vi "Joystick and Camera.vi"() -> ()   [LabVIEW 2020]
uses:
  Classes/Controller/Camera/Camera.lvclass
  Classes/Controller/Controller.lvclass
  Classes/Controller/I-O/I-O.lvclass
  Classes/Controller/Motion/A3200/A3200.lvclass
  Classes/Controller/Motion/Motion.lvclass
  Classes/Controller/Camera/Machine Vision.ctl
  Classes/Controller/Camera/Camera settings.ctl
  Classes/Controller/Camera/Image processing.ctl
  Classes/Controller/Camera/Material.ctl
panel:
  in  "Find fiducial":bool
  in  "Loop count":dbl=1.0
  in  "X, Y pixel stride":dbl[](array[numeric])=[1520.0, 2160.0]
  in  "Draw spiral":bool
  out "Move by":dbl[](array[numeric])
  in  "Find in Image":bool
  in  "Screen Grab":bool
  in  "Focus step size":dbl format="%#_13g"
  in  "number of focus steps":i32
  out "Radius (Real-World)":dbl
  out "error out":errorcluster
  in  "Find fiducial center":bool
  out "Average Strength":dbl
  in  "Focus":bool
  in  "Material":T1
  in  "Override presets":bool
  in  "Camera settings":T2={"Gamma"=1.6, "Gain"=0, "Sharpness"=0, "Contrast"=0.0, "Exposure"=0.0078125} {"Exposure" min=0.000244140625 max=0.5 scale=0.0002..0.5; "Contrast" min=0.0 max=1.0 scale=0.0..1.0; "Sharpness" min=0 max=2 step=1 scale=0.0..2.0; "Gain" min=0 max=100 step=1 scale=0.0..100.0; "Gamma" min=0.01 max=10.0 scale=0.01..10.0}
  in  "Image processing":T3={"Brightness"=128.0, "Contrast"=45.0, "Gamma"=1.0471123} {"Brightness" scale=0.0..400.0; "Contrast" scale=0.0..90.0; "Gamma" scale=0.005..5.0}
  out "XYZTheta Out":dbl[](array[numeric])
  in  "Machine Vision":T4
  in  "Move 10cm Right":bool
  in  "Move 10cm Backward":bool
  in  "Move 10cm Forward":bool
  in  "Move 10cm Left":bool
  in  "Record Measurement":bool=TRUE
  in  "Dismount Silicon Tray":bool
  in  "Secure Silicon Tray":bool
  in  "Z Go":bool
  in  "Position":dbl
  in  "XYZTheta":dbl[](array[numeric])
  in  "Go":bool
  in  "Joystick":bool
  out "Sum":dbl[](array[numeric]) format="%#.6g"
  out "Gantry":dbl[](array[numeric]) format="%#.6g"
  in  "Stop":bool
  out "Image":T5(plugin-control)
  out "Camera":dbl[](array[numeric])
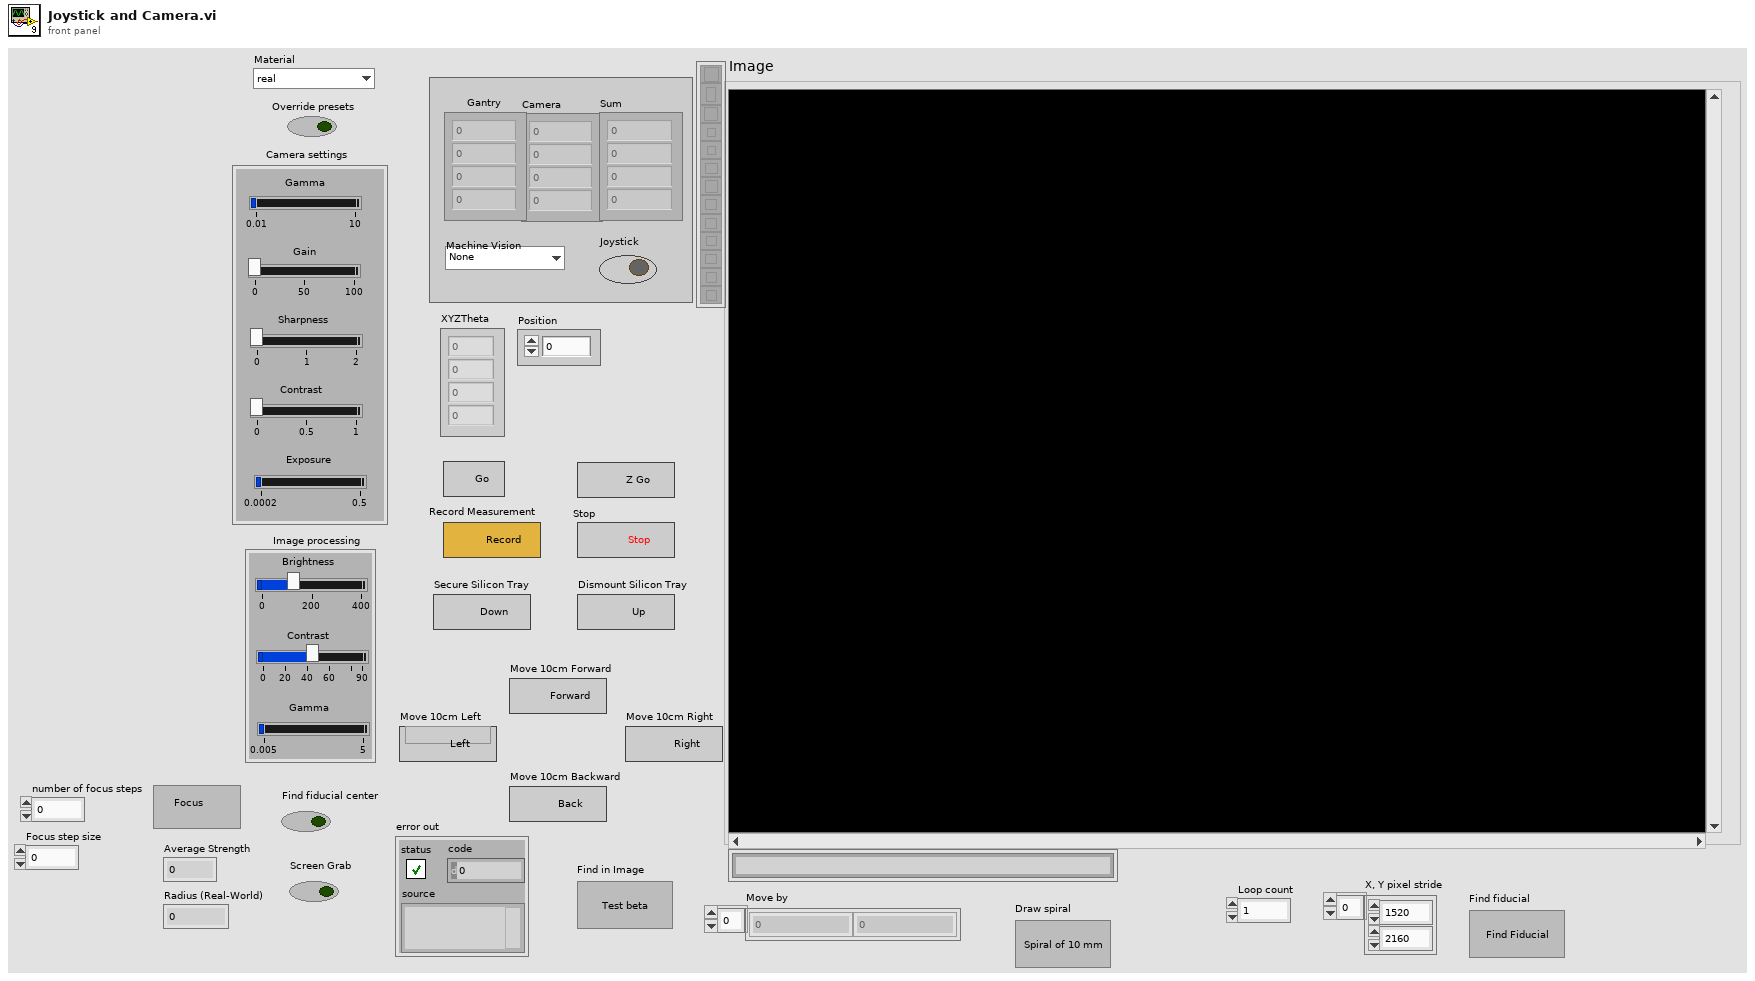
[diagram p1: front panel]
types:
  T1 = typedef "Camera.lvclass/Material.ctl" = enum16{"real", "dummy", "PETG"}
  T2 = typedef "Camera.lvclass/Camera settings.ctl" = cluster{"Gamma":dbl, "Gain":i64, "Sharpness":i64, "Contrast":dbl, "Exposure":dbl}
  T3 = typedef "Camera.lvclass/Image processing.ctl" = cluster{"Brightness":sgl, "Contrast":sgl, "Gamma":sgl}
  T4 = typedef "Camera.lvclass/Machine Vision.ctl" = enum16{"None", "Tray Fiducials", "HPK Silicon", "100um dot", "Hexaboard", "Corner (TL, BR)", "Corner (BL, TR)", "BP gold pad 1", "BP gold pad 2", "BP gold pad 3", "dummy sensor CH2", "dummy sensor CH7", "dummy sensor CH191", "dummy sensor CH197", "sensor box", "sensor circle", "PCB PETG CH2", "PCB PETG CH7", "PCB PETG CH191", "PCB PETG CH197"}
  T5 = typedef "IMAQ Image.ctl" = refnum<image>
  T6 = enum16{"open", "replace", "create", "open or create", "replace or create", "replace or create with confirmation"}
  T7 = typedef "Controller.lvclass/Controllers.ctl" = cluster{"I-O.lvclass":refnum<class "I-O.lvclass">, "Gantry":refnum<k24>, "Dispenser":refnum<visa-resource-name>}
  T8 = typedef "I-O.lvclass/Pin Map.ctl" = cluster{"Region Valves":i32[], "Extra Valves":dbl[][][], "Tool Primary Valve":i32, "Tool Secondary Valve":i32, "Region Sensors":i32[], "Extra Sensors":dbl[][][], "Tool Primary Sensor":dbl, "Tool Secondary Sensor":dbl, "Compression Sensor":dbl, "5V":i32, "Dispenser Sensor":dbl}
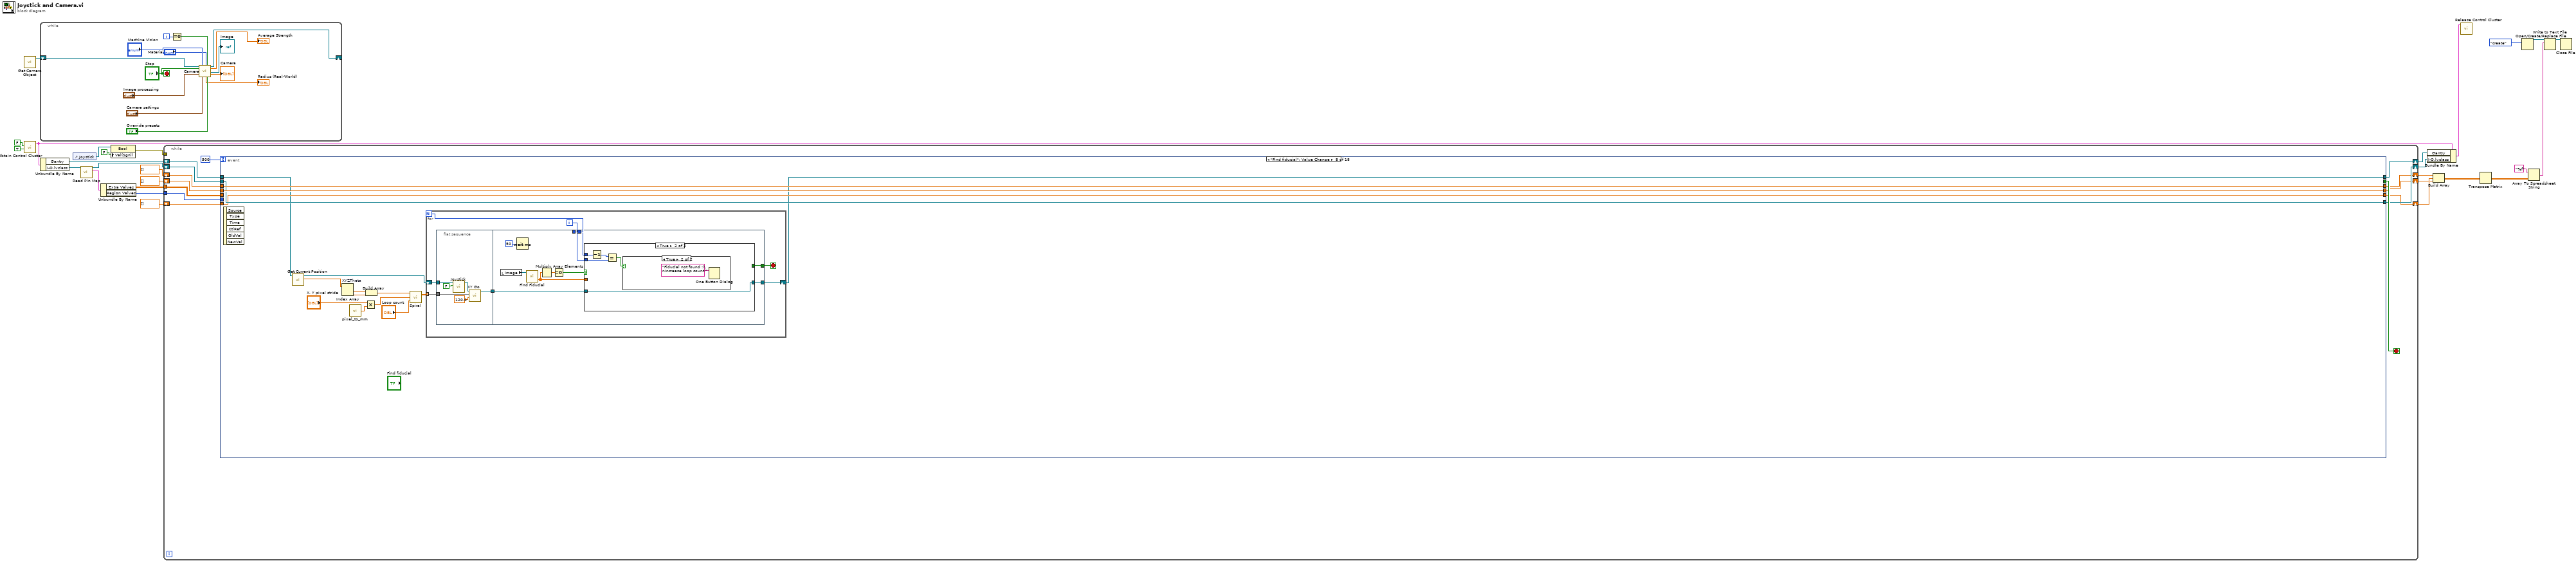
[diagram p0: block diagram]
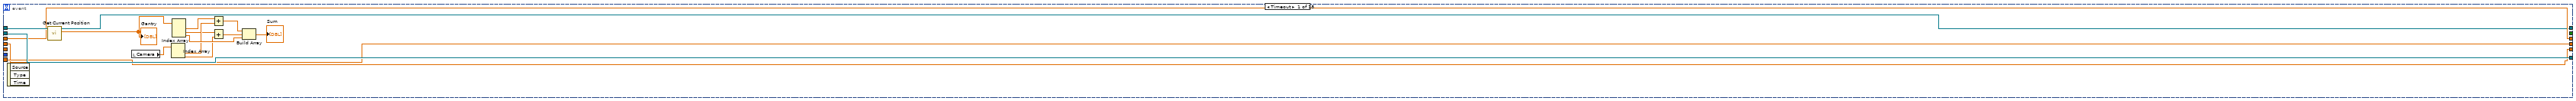
[diagram p2: hidden frame]
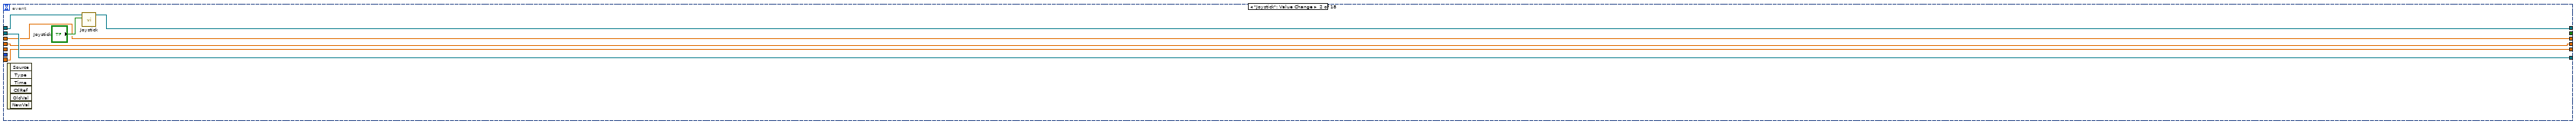
[diagram p3: hidden frame]
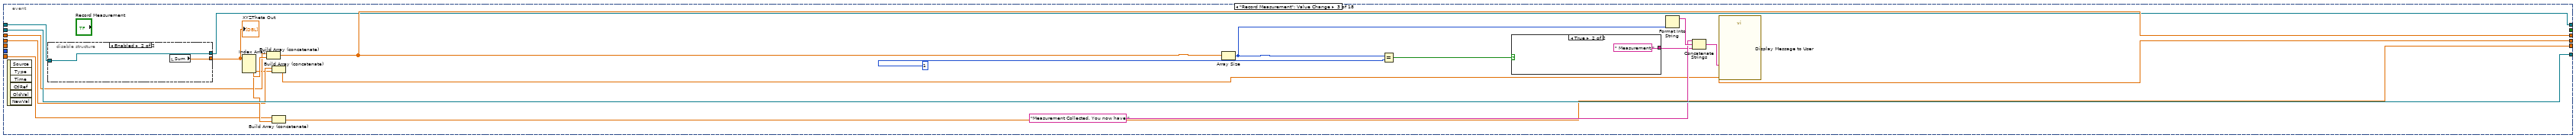
[diagram p4: hidden frame]
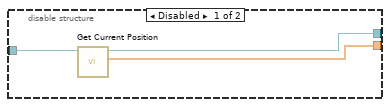
[diagram p5: hidden frame]
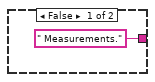
[diagram p6: hidden frame]
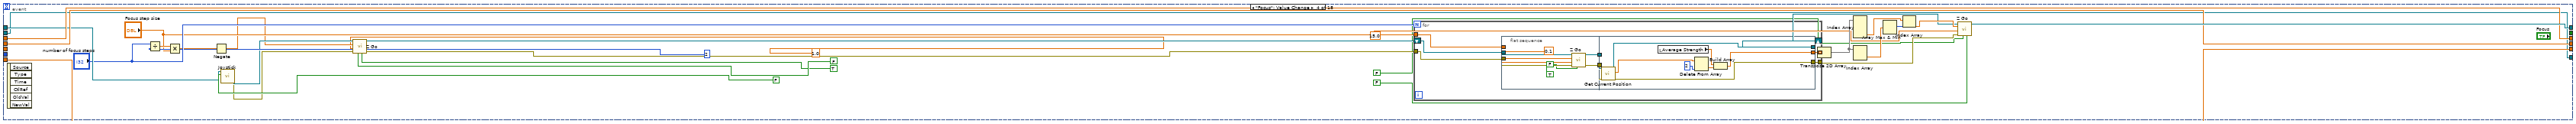
[diagram p7: hidden frame]
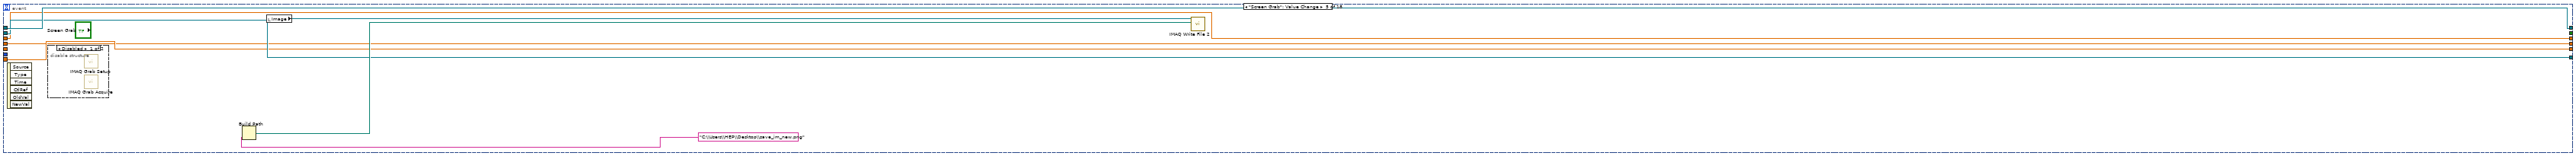
[diagram p8: hidden frame]
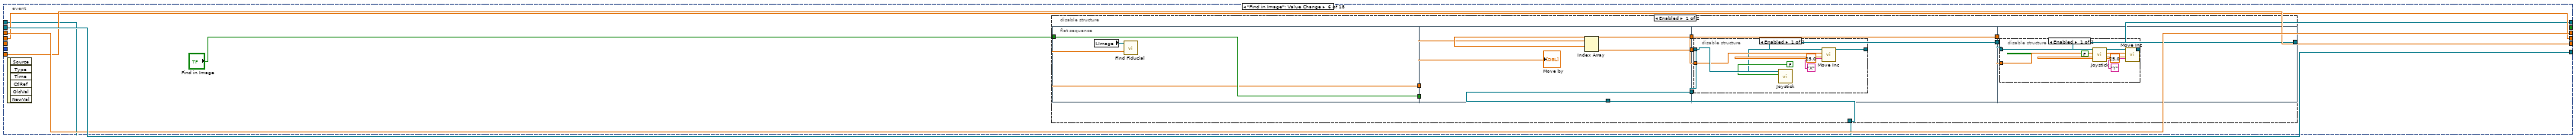
[diagram p10: hidden frame]
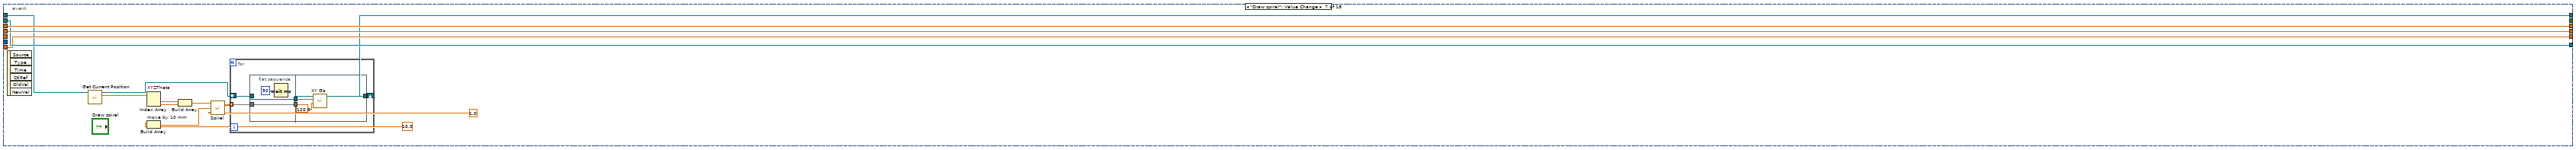
[diagram p14: hidden frame]
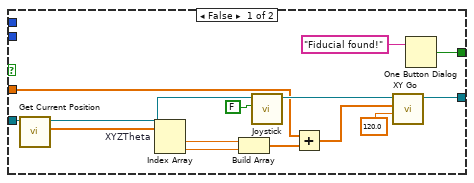
[diagram p15: hidden frame]
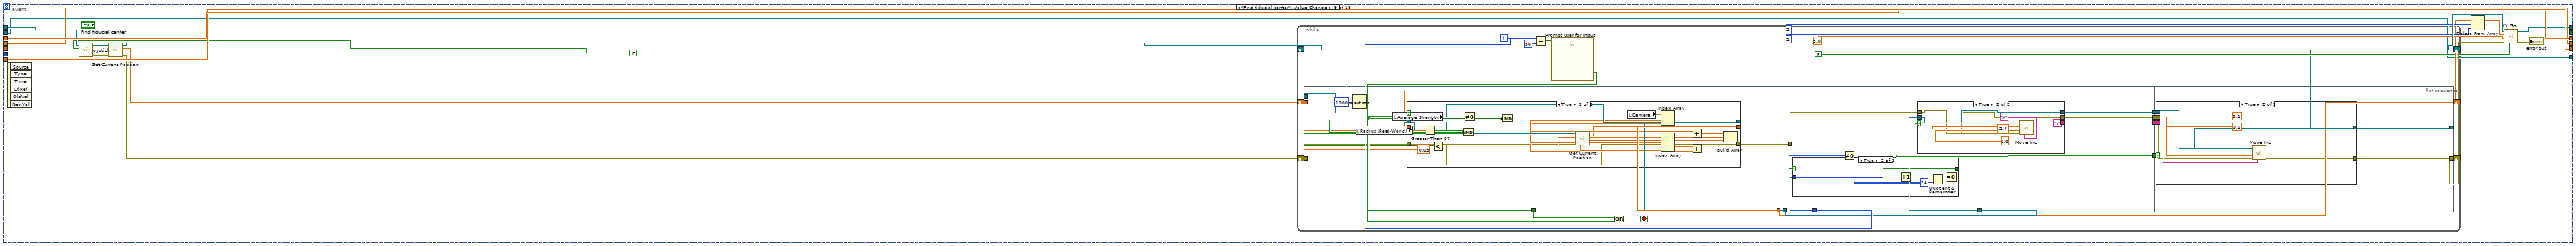
[diagram p17: hidden frame]
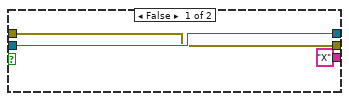
[diagram p20: hidden frame]
diagram:
  n1 = call "Get Camera Object.vi"() -> ("Camera out"=w23:refnum<class "Camera.lvclass">)  [unwired: 10 in, 1 out]
  n2 = call "Obtain Control Cluster.vi"("I/O"=TRUE, "Dispense"=FALSE) -> ("Control Out"=w1:T7)  [unwired: 9 in]
  n3 = while {
    shift-right: [w42] -> _
    shift-left: w23 -> [w43]
    i -> [w34]
    stop <- "Stop" stop-if-true
    n4 = Equal To 0?(x=w34) -> (x = 0?=w33:bool)
    n5 = call "Camera.vi"("Camera in"=w43, "Stop"="Stop", "BCG Image Processing"="Image processing", "Machine Vision"="Machine Vision", "Camera settings"="Camera settings", "Material"="Material", "Loop 0"=w33, "Override presets"="Override presets") -> ("Radius (Real-World)"=→"Radius (Real-World)":dbl, "Camera out"=w42:refnum<class "Camera.lvclass">, "Average Strength"=→"Average Strength":dbl, "Image"=→"Image":T5, "Camera"=→"Camera":dbl[])  [unwired: 6 in, 1 out]
  }
  n6 = Unbundle By Name(w1) -> ("Gantry"=w24:refnum<k24>, "I-O.lvclass"=w22:refnum<class "I-O.lvclass">)
  n7 = control-ref of="Joystick"() -> (w28:refnum<vi>)
  n8 = call-dynamic "Read Pin Map.vi"("I-O in"=w22) -> ("Pin Map 2"=w20:T8, "I-O out"=w21:refnum<class "I-O.lvclass">)  [unwired: 8 in, 1 out]
  n9 = Unbundle By Name(w20) -> ("Extra Valves"=w18:dbl[][][], "Region Valves"=w19:i32[])
  n10 = property class="Bool"(reference=w28, "Val(Sgnl)"=FALSE ("Value (Signaling)")) -> (error out=w27:errorcluster)  [unwired: 1 in, 1 out]
  n11 = while {
    shift-right: [w44] -> w4
    shift-left: w24 -> [w55]
    tunnel: w27 -> [_]
    shift-right: [w53] -> w3
    shift-left: w21 -> [w54]
    tunnel: w19 -> [w52]
    tunnel: w18 -> [w51]
    shift-right: [w46] -> w6
    shift-left: dbl[] [] -> [w50]
    shift-right: [w48] -> w7
    shift-left: dbl[] [] -> [w49]
    shift-right: [w45] -> w8
    shift-left: dbl[] [] -> [w47]
    stop <- w56 stop-if-true
    n12 = event shown="[7] \"Find fiducial\": Value Change" {
      selector: _ -> [_ _ _ _ _ _ _ _ _ _ _ _ _ _ _ _ _ _]
      dyn-events: _ -> [_ _ _ _ _ _ _ _ _ _ _ _ _ _ _ _ _ _]
      timeout: 500 -> [_ _ _ _ _ _ _ _ _ _ _ _ _ _ _ _ _ _]
      tunnel: [_ _ _ _ _ _ _ _ _ _ _ _ _ _ _ _ _ TRUE] -> w56
      tunnel: w55 -> [w73 w80 w83 w124 w169 w174 w228 w257 w323 w442 w453 w464 w475 w477 w487 w504 w523 w531]
      tunnel: w54 -> [w72 w78 w100 w108 w168 w178 w231 w260 w306 w437 w449 w461 w472 w484 w496 w501 w520 w529]
      tunnel: [w72 w78 w100 w108 w168 w178 w231 w260 w306 w437 w449 w461 w472 w481 w491 w501 w520 w529] -> w53
      tunnel: w52 -> [_ _ _ _ _ _ _ _ _ _ _ _ _ w486 w495 _ _ _]
      tunnel: w51 -> [_ _ _ _ _ _ _ _ _ _ _ _ _ _ _ _ _ _]
      tunnel: w50 -> [w71 w77 w87 w127 w166 w176 w230 w259 w325 w440 w452 w463 w474 w480 w490 w500 w519 w528]
      tunnel: [w71 w77 w91 w127 w166 w176 w230 w259 w325 w440 w452 w463 w474 w480 w490 w500 w519 w528] -> w46
      tunnel: w49 -> [w70 w76 w88 w128 w167 w177 w233 w262 w326 w439 w451 w462 w473 w479 w489 w499 w518 w527]
      tunnel: [w70 w76 w90 w128 w167 w177 w233 w262 w326 w439 w451 w462 w473 w479 w489 w499 w518 w527] -> w48
      tunnel: w47 -> [w69 w75 w86 w126 w165 w175 w232 w261 w324 w438 w450 w460 w471 w478 w488 w498 w517 w526]
      tunnel: [w69 w75 w84 w126 w165 w175 w232 w261 w324 w438 w450 w460 w471 w478 w488 w498 w517 w526] -> w45
      tunnel: [w68 w74 w81 w129 w169 w173 w229 w258 w320 w436 w445 w455 w467 w477 w487 w497 w516 w524] -> w44
      event Timeout {
        n13 = event-data() -> ()  [unwired: 1 in, 3 out]
        n14 = call "Get Current Position.vi"("Gantry In"=w73) -> ("XYZTheta Out"=w65:dbl[], "Gantry Out"=w68:refnum<k24>)  [unwired: 8 in, 1 out]
        "Gantry" <- w65
        n15 = local read "Camera"() -> (w62:dbl[])
        n16 = Index Array(array=w62) -> (element #1=w61:dbl, element #2=w58:dbl)  [unwired: 2 in]
        n17 = Index Array(array=w65) -> (element #1=w63:dbl, element #2=w59:dbl, element #3=w66:dbl)  [unwired: 3 in]
        n18 = Add(x=w63, y=w61) -> (x+y=w64:dbl)
        n19 = Add(x=w59, y=w58) -> (x+y=w60:dbl)
        n20 = Build Array(w64, w60, w66) -> (→"Sum":dbl[])
      }
      event "Joystick": Value Change {
        n21 = event-data() -> ()  [unwired: 1 in, 6 out]
        n22 = call "Joystick.vi"("Joystick"="Joystick", "Gantry In"=w80) -> ("Gantry Out"=w74:refnum<k24>)  [unwired: 8 in, 1 out]
      }
      event "Record Measurement": Value Change {
        n23 = event-data() -> ()  [unwired: 1 in, 6 out]
        n24 = disable-structure shown="Enabled" {
          disable-tunnel: [w102 w104] -> w82
          disable-tunnel: w83 -> [w103 w105]
          disable-tunnel: [w101 w105] -> w81
          frame Disabled {
            n25 = call "Get Current Position.vi"("Gantry In"=w103) -> ("XYZTheta Out"=w102:dbl[], "Gantry Out"=w101:refnum<k24>)  [unwired: 8 in, 1 out]
          }
          frame Enabled {
            n26 = local read "Sum"() -> (w104:dbl[])
          }
        }
        "XYZTheta Out" <- w82
        n27 = Index Array(array=w82) -> (element #1=w99:dbl, element #2=w89:dbl, element #3=w85:dbl)  [unwired: 3 in]
        n28 = Build Array (concatenate) "Build Array"(w88, w99) -> (w90:dbl[])
        n29 = Build Array (concatenate)(w86, w85) -> (w84:dbl[])
        n30 = Build Array (concatenate)(w87, w89) -> (w91:dbl[])
        n31 = Array Size(array=w90) -> (size(s)=w94:i32)
        n32 = Equal?(x=w94, y=1) -> (x = y?=w93:bool)
        n33 = case shown="True" w93 {
          tunnel: [" Measurements." " Measurement."] -> w92
          frame False {
          }
          frame True {
          }
        }
        n34 = Format Into String(w94) -> (resulting string=w98:string)  [unwired: 3 in, 1 out]
        n35 = Concatenate Strings("Measurement Collected. You now have ", w98, w92) -> (w96:string)
        n36 = call "Display Message to User"("Message"=w96) -> ()  [unwired: 9 in, 2 out]
      }
      event "Focus": Value Change {
        n37 = event-data() -> ()  [unwired: 1 in, 6 out]
        n38 = Divide(x="number of focus steps", y=2) -> (x/y=w121:dbl)
        n39 = Multiply(x=w121, y="Focus step size") -> (x*y=w119:dbl)
        n40 = Negate(x=w119) -> (-x=w114:dbl)
        n41 = call "Joystick.vi"("Joystick"=FALSE, "Gantry In"=w124) -> ("error out"=w115:errorcluster, "Gantry Out"=w118:refnum<k24>)  [unwired: 8 in]
        n42 = call "Z Go.vi"("Increment"=TRUE, "Return Immediately"=FALSE ("Increment"), "error in (no error)"=w115, "Speed In"=1.0 ("Speed"), "Position In"=w114, "Gantry In"=w118) -> ("error out"=w116:errorcluster, "Gantry Out"=w117:refnum<k24>)  [unwired: 2 in, 2 out]
        n43 = for {
          N: "number of focus steps" -> [_]
          tunnel: [w143] -> w137 mode=indexing
          tunnel: w116 -> [w142]
          tunnel: [w140] -> w130
          shift-right: [w144] -> w131
          shift-left: w117 -> [w146]
          tunnel: "Focus step size" -> [w139]
          n44 = flat-sequence {
            tunnel: w146 -> [w153]
            tunnel: [w152] -> w145
            tunnel: w142 -> [w151]
            tunnel: [w150] -> w141
            tunnel: w139 -> [w149]
            tunnel: w145 -> [w163]
            tunnel: [w162] -> w144
            tunnel: [w161] -> w143
            tunnel: w141 -> [w157]
            tunnel: [w156] -> w140
            frame #0 {
              n45 = call "Z Go.vi"("Increment"=TRUE, "Return Immediately"=FALSE ("Increment"), "error in (no error)"=w151, "Speed In"=0.1 ("Speed"), "Position In"=w149, "Gantry In"=w153) -> ("error out"=w150:errorcluster, "Gantry Out"=w152:refnum<k24>)  [unwired: 2 in, 2 out]
            }
            frame #1 {
              n46 = call "Get Current Position.vi"("error in (no error)"=w157, "Gantry In"=w163) -> ("error out"=w156:errorcluster, "XYZTheta Out"=w160:dbl[], "Gantry Out"=w162:refnum<k24>)  [unwired: 7 in]
              n47 = local read "Average Strength"() -> (w155:dbl)
              n48 = Delete From Array(array=w160, index=2) -> (deleted portion=w158:dbl)  [unwired: 1 in, 1 out]
              n49 = Build Array(w155, w158) -> (w161:dbl[])
            }
          }
        }
        n50 = Transpose 2D Array(2D array=w137) -> (transposed array=w136:dbl[][])
        n51 = Index Array(array=w136) -> (element #2=w135:dbl[])  [unwired: 4 in, 1 out]
        n52 = Index Array(array=w136) -> (element=w138:dbl[])  [unwired: 2 in]
        n53 = Array Max & Min(array=w138) -> (max index (indices)=w134:i32)  [unwired: 3 out]
        n54 = Index Array(array=w135, index=w134) -> (element=w133:dbl)
        n55 = call "Z Go.vi"("Increment"=FALSE, "Return Immediately"=FALSE ("Increment"), "error in (no error)"=w130, "Speed In"=15.0 ("Speed"), "Position In"=w133, "Gantry In"=w131) -> ("Gantry Out"=w129:refnum<k24>)  [unwired: 2 in, 3 out]
      }
      event "Screen Grab": Value Change {
        n56 = event-data() -> ()  [unwired: 1 in, 6 out]
        n57 = disable-structure shown="Disabled" {
          frame Disabled {
            n58 = call <vilib>:"IMAQ Grab Setup.vi"() -> ()  [unwired: 10 in, 2 out]
            n59 = call <vilib>:"IMAQ Grab Acquire.vi"() -> ()  [unwired: 8 in, 4 out]
          }
          frame Enabled {
          }
        }
        n60 = Build Path(name or relative path="C:\\Users\\HEP\\Desktop\\save_im_new.png") -> (appended path=w171:path)  [unwired: 1 in]
        n61 = local read "Image"() -> (w164:T5)
        n62 = call-poly "IMAQ Write File 2"("File Path"=w171, "Image"=w164) -> ()  [unwired: 8 in, 2 out]
      }
      event "Find in Image": Value Change {
        n63 = event-data() -> ()  [unwired: 1 in, 6 out]
        n64 = disable-structure shown="Enabled" {
          disable-tunnel: w174 -> [w182 w219]
          disable-tunnel: [w181 w219] -> w173
          disable-tunnel: "Find in Image" -> [w180 _]
          frame Enabled {
            n65 = flat-sequence {
              tunnel: [w191] -> w188
              tunnel: w180 -> [w191]
              tunnel: [w190] -> w179
              tunnel: w188 -> [_]
              tunnel: w182 -> [w195]
              tunnel: [w195] -> w187
              tunnel: [w194] -> w186
              tunnel: [w193] -> w185
              tunnel: w179 -> [w192]
              tunnel: w187 -> [w199]
              tunnel: [w198] -> w184
              tunnel: w186 -> [w197]
              tunnel: [w196] -> w183
              tunnel: w185 -> [w196]
              tunnel: [w209] -> w181
              tunnel: w184 -> [w210]
              tunnel: w183 -> [w208]
              frame #0 {
                n66 = local read "Image"() -> (w189:T5)
                n67 = call "Find Fiducial.vi"("Image"=w189) -> ("Move by (mm)"=w190:dbl[])  [unwired: 3 in]
              }
              frame #1 {
                n68 = Index Array(array=w192) -> (element #1=w194:dbl, element #2=w193:dbl)  [unwired: 2 in]
                "Move by" <- w192
              }
              frame #2 {
                n69 = disable-structure shown="Enabled" {
                  disable-tunnel: w199 -> [w206 w207]
                  disable-tunnel: [w205 w207] -> w198
                  disable-tunnel: w197 -> [w204 _]
                  frame Enabled {
                    n70 = call "Joystick.vi"("Joystick"=FALSE, "Gantry In"=w206) -> ("Gantry Out"=w200:refnum<k24>)  [unwired: 8 in, 1 out]
                    n71 = call "Move Inc.vi"("Axis"="X", "Speed"=25.0, "Distance"=w204, "Gantry In"=w200) -> ("Gantry Out"=w205:refnum<k24>)  [unwired: 6 in, 1 out]
                  }
                  frame Disabled {
                  }
                }
              }
              frame #3 {
                n72 = disable-structure shown="Enabled" {
                  disable-tunnel: w210 -> [w217 w218]
                  disable-tunnel: [w216 w218] -> w209
                  disable-tunnel: w208 -> [w215 _]
                  frame Enabled {
                    n73 = call "Joystick.vi"("Joystick"=FALSE, "Gantry In"=w217) -> ("Gantry Out"=w211:refnum<k24>)  [unwired: 8 in, 1 out]
                    n74 = call "Move Inc.vi"("Axis"="Y", "Speed"=25.0, "Distance"=w215, "Gantry In"=w211) -> ("Gantry Out"=w216:refnum<k24>)  [unwired: 6 in, 1 out]
                  }
                  frame Disabled {
                  }
                }
              }
            }
          }
          frame Disabled {
          }
        }
      }
      event "Draw spiral": Value Change {
        w221 = 10.0 ("element")
        n75 = event-data() -> ()  [unwired: 1 in, 6 out]
        n76 = call "Get Current Position.vi"("Gantry In"=w228) -> ("XYZTheta Out"=w226:dbl[], "Gantry Out"=w227:refnum<k24>)  [unwired: 8 in, 1 out]
        n77 = Index Array "XYZTheta"(array=w226) -> (element #1=w225:dbl, element #2=w224:dbl)  [unwired: 2 in]
        n78 = Build Array "move by 10 mm"(w221, w221) -> (w220:dbl[])
        n79 = Build Array(w225, w224) -> (w223:dbl[])
        n80 = call "Spiral.vi"("Loop count"=1.0, "X, Y stride (mm)"=w220, "XY center (mm)"=w223) -> ("Spiral coordinates"=w234:dbl[][])  [unwired: 1 in]
        n81 = for {
          tunnel: w234 -> [w239] mode=indexing
          shift-right: [w237] -> w229
          shift-left: w227 -> [w238]
          n82 = flat-sequence {
            tunnel: w238 -> [w241]
            tunnel: w239 -> [w242]
            tunnel: [w242] -> w236
            tunnel: [w241] -> w235
            tunnel: [w243] -> w237
            tunnel: w236 -> [w245]
            tunnel: w235 -> [w244]
            frame #0 {
              n83 = Wait (ms)(milliseconds to wait=u32 50) -> ()  [unwired: 1 out]
            }
            frame #1 {
              n84 = call "XY Go.vi"("Speed"=120.0, "XY In"=w245, "Gantry In"=w244) -> ("Gantry Out"=w243:refnum<k24>)  [unwired: 6 in, 2 out]
            }
          }
        }
      }
      event "Find fiducial": Value Change {
        n85 = event-data() -> ()  [unwired: 1 in, 6 out]
        n86 = call "Get Current Position.vi"("Gantry In"=w257) -> ("XYZTheta Out"=w255:dbl[], "Gantry Out"=w256:refnum<k24>)  [unwired: 8 in, 1 out]
        n87 = Index Array "XYZTheta"(array=w255) -> (element #1=w254:dbl, element #2=w253:dbl)  [unwired: 2 in]
        n88 = call "pixel_to_mm.vi"() -> ("mm/pixel"=w250:dbl)  [unwired: 2 in]
        n89 = Multiply(x="X, Y pixel stride", y=w250) -> (x*y=w249:dbl[])
        n90 = Build Array(w254, w253) -> (w252:dbl[])
        n91 = call "Spiral.vi"("Loop count"="Loop count", "X, Y stride (mm)"=w249, "XY center (mm)"=w252) -> ("Spiral coordinates"=w247:dbl[][])  [unwired: 1 in]
        n92 = for {
          N -> [w265]
          tunnel: w247 -> [w269] mode=indexing
          shift-right: [w267] -> w258
          shift-left: w256 -> [w268]
          i -> [w264]
          stop <- w266 stop-if-true
          n93 = flat-sequence {
            tunnel: [w270] -> w263
            tunnel: w268 -> [w272]
            tunnel: w269 -> [w271]
            tunnel: [w282] -> w267
            tunnel: [w284] -> w266
            tunnel: w265 -> [w281]
            tunnel: w264 -> [w280]
            tunnel: w263 -> [w279]
            frame #0 {
              n94 = call "Joystick.vi"("Joystick"=FALSE, "Gantry In"=w272) -> ("Gantry Out"=w275:refnum<k24>)  [unwired: 8 in, 1 out]
              n95 = call "XY Go.vi"("Speed"=120.0, "XY In"=w271, "Gantry In"=w275) -> ("Gantry Out"=w270:refnum<k24>)  [unwired: 6 in, 2 out]
            }
            frame #1 {
              n96 = local read "Image"() -> (w285:T5)
              n97 = Wait (ms)(milliseconds to wait=u32 50) -> ()  [unwired: 1 out]
              n98 = call "Find Fiducial.vi"("Image"=w285) -> ("Move by (mm)"=w283:dbl[])  [unwired: 3 in]
              n99 = Multiply Array Elements(1:w283) -> (0:w277:dbl)
              n100 = Equal To 0?(x=w277) -> (x = 0?=w276:bool)
              n101 = case shown="True" w276 {
                tunnel: [w289 _] -> w284
                tunnel: w283 -> [w288 _]
                tunnel: [w287 w300] -> w282
                tunnel: w281 -> [_ w302]
                tunnel: w280 -> [_ w301]
                tunnel: w279 -> [w286 w300]
                frame False {
                  n102 = call "Get Current Position.vi"("Gantry In"=w286) -> ("XYZTheta Out"=w294:dbl[], "Gantry Out"=w299:refnum<k24>)  [unwired: 8 in, 1 out]
                  n103 = Index Array "XYZTheta"(array=w294) -> (element #1=w295:dbl, element #2=w296:dbl)  [unwired: 2 in]
                  n104 = Build Array(w295, w296) -> (w297:dbl[])
                  n105 = call "Joystick.vi"("Joystick"=FALSE, "Gantry In"=w299) -> ("Gantry Out"=w293:refnum<k24>)  [unwired: 8 in, 1 out]
                  n106 = Add(x=w288, y=w297) -> (x+y=w298:dbl[])
                  n107 = call "XY Go.vi"("Speed"=120.0, "XY In"=w298, "Gantry In"=w293) -> ("Gantry Out"=w287:refnum<k24>)  [unwired: 6 in, 2 out]
                  n108 = One Button Dialog(message="Fiducial found!") -> (true=w289:bool)  [unwired: 1 in]
                }
                frame True {
                  n109 = Decrement(x=w302) -> (x-1=w304:i32)
                  n110 = Equal?(x=w304, y=w301) -> (x = y?=w303:bool)
                  n111 = case shown="True" w303 {
                    frame False {
                    }
                    frame True {
                      n112 = One Button Dialog(message="Fiducial not found :(\nIncrease loop count.") -> ()  [unwired: 1 in, 1 out]
                    }
                  }
                }
              }
            }
          }
        }
      }
      event "Find fiducial center": Value Change {
        n113 = event-data() -> ()  [unwired: 1 in, 6 out]
        n114 = call "Joystick.vi"("Joystick"=FALSE, "Gantry In"=w323) -> ("error out"=w312:errorcluster, "Gantry Out"=w314:refnum<k24>)  [unwired: 8 in]
        n115 = call "Get Current Position.vi"("error in (no error)"=w312, "Gantry In"=w314) -> ("error out"=w311:errorcluster, "XYZTheta Out"=w309:dbl[], "Gantry Out"=w313:refnum<k24>)  [unwired: 7 in]
        n116 = while {
          shift-right: [w343] -> w321
          shift-left: w313 -> [w332]
          shift-right: [w344] -> w319
          shift-left: w311 -> [w329]
          shift-right: [w327] -> w308
          shift-left: w309 -> [w330]
          i -> [w338]
          stop <- w336 stop-if-true
          n117 = flat-sequence {
            tunnel: [w356] -> w333
            tunnel: [w355] -> w327
            tunnel: w332 -> [w354]
            tunnel: [w353] -> w331
            tunnel: w330 -> [w352]
            tunnel: w329 -> [w351]
            tunnel: [w350] -> w328
            tunnel: w338 -> [w384]
            tunnel: [w383] -> w342
            tunnel: [w382] -> w341
            tunnel: w331 -> [w381]
            tunnel: [w380] -> w340
            tunnel: [w379] -> w339
            tunnel: w328 -> [w377]
            tunnel: [w405] -> w343
            tunnel: [w406] -> w344
            tunnel: w342 -> [w407]
            tunnel: w341 -> [w404]
            tunnel: w340 -> [w403]
            tunnel: w339 -> [w402]
            frame #0 {
              n118 = Wait (ms)(milliseconds to wait=u32 1000) -> ()  [unwired: 1 out]
              n119 = local read "Radius (Real-World)"() -> (w346:dbl)
              n120 = local read "Average Strength"() -> (w359:dbl)
              n121 = Greater Than 0?(x=w346) -> (x > 0?=w348:bool)
              n122 = Less?(x=w346, y=0.05) -> (x < y?=w347:bool)
              n123 = And(x=w348, y=w347) -> (x .and. y?=w357:bool)
              n124 = Not Equal To 0?(x=w359) -> (x != 0?=w358:bool)
              n125 = And(x=w358, y=w357) -> (x .and. y?=w356:bool)
              n126 = case shown="True" w356 {
                tunnel: [w361 w365] -> w355
                tunnel: w354 -> [w362 w376]
                tunnel: [w362 w375] -> w353
                tunnel: w352 -> [w361 _]
                tunnel: w351 -> [w360 w364]
                tunnel: [w360 w363] -> w350
                frame False {
                }
                frame True {
                  n127 = call "Get Current Position.vi"("error in (no error)"=w364, "Gantry In"=w376) -> ("error out"=w363:errorcluster, "XYZTheta Out"=w374:dbl[], "Gantry Out"=w375:refnum<k24>)  [unwired: 7 in]
                  n128 = local read "Camera"() -> (w372:dbl[])
                  n129 = Index Array(array=w372) -> (element #1=w369:dbl, element #2=w368:dbl)  [unwired: 2 in]
                  n130 = Index Array(array=w374) -> (element #1=w373:dbl, element #2=w370:dbl, element #3=w371:dbl)  [unwired: 3 in]
                  n131 = Add(x=w373, y=w369) -> (x+y=w367:dbl)
                  n132 = Add(x=w370, y=w368) -> (x+y=w366:dbl)
                  n133 = Build Array(w367, w366, w371) -> (w365:dbl[])
                }
              }
            }
            frame #1 {
              n134 = Not Equal To 0?(x=w384) -> (x != 0?=w382:bool)
              n135 = case shown="True" w382 {
                selector: w382 -> [w385 _]
                tunnel: [w385 w389] -> w378
                tunnel: w384 -> [_ w387]
                frame False {
                }
                frame True {
                  n136 = Increment(x=w387) -> (x+1=w386:i32)
                  n137 = Quotient & Remainder(x=w386, y=24) -> (x-y*floor(x/y)=w388:i32)  [unwired: 1 out]
                  n138 = Equal To 0?(x=w388) -> (x = 0?=w389:bool)
                }
              }
              n139 = case shown="True" w378 {
                tunnel: ["X" ("Axis") "Y" ("Axis")] -> w383
                tunnel: w381 -> [w392 w400]
                tunnel: [w392 w399] -> w380
                tunnel: [w391 w395] -> w379
                tunnel: w377 -> [w391 w394]
                frame False {
                }
                frame True {
                  n140 = call "Move Inc.vi"("Axis"="X", "error in (no error)"=w394, "Speed"=1.0, "Distance"=-2.4, "Gantry In"=w400) -> ("error out"=w395:errorcluster, "Gantry Out"=w399:refnum<k24>)  [unwired: 5 in]
                }
              }
            }
            frame #2 {
              n141 = case shown="True" w404 {
                tunnel: w407 -> [_ w432]
                tunnel: w402 -> [w408 w431]
                tunnel: w403 -> [w411 w429]
                tunnel: [w409 w428] -> w406
                tunnel: [w410 w427] -> w405
                frame False {
                  n142 = disable-structure shown="Enabled" {
                    disable-tunnel: w411 -> [w423 w425]
                    disable-tunnel: [w421 w425] -> w410
                    disable-tunnel: [w420 w424] -> w409
                    disable-tunnel: w408 -> [w418 w424]
                    frame Enabled {
                      n143 = call "Move Inc.vi"("Axis"="X", "error in (no error)"=w418, "Speed"=1.0, "Distance"=-0.8, "Gantry In"=w423) -> ("error out"=w419:errorcluster, "Gantry Out"=w422:refnum<k24>)  [unwired: 5 in]
                      n144 = call "Move Inc.vi"("Axis"="Y", "error in (no error)"=w419, "Speed"=1.0, "Distance"=-1.0, "Gantry In"=w422) -> ("error out"=w420:errorcluster, "Gantry Out"=w421:refnum<k24>)  [unwired: 5 in]
                    }
                    frame Disabled {
                    }
                  }
                }
                frame True {
                  n145 = call "Move Inc.vi"("Axis"=w432, "error in (no error)"=w431, "Speed"=0.1, "Distance"=0.1, "Gantry In"=w429) -> ("error out"=w428:errorcluster, "Gantry Out"=w427:refnum<k24>)  [unwired: 5 in]
                }
              }
            }
          }
          n146 = Equal?(x=w338, y=50) -> (x = y?=w335:bool)
          n147 = call "Prompt User for Input"("Enable"=w335) -> ("OK"=w334:bool)  [unwired: 17 in, 1 out]
          n148 = Or(x=w333, y=w334) -> (x .or. y?=w336:bool)
        }
        n149 = Delete From Array(array=w308, length=2, index=2) -> (array with subset deleted=w316:dbl[])  [unwired: 1 out]
        n150 = call "XY Go.vi"("return immediately"=FALSE, "error in (no error)"=w319, "Speed"=5.0, "XY In"=w316, "Gantry In"=w321) -> ("error out"=→"error out":errorcluster, "Gantry Out"=w320:refnum<k24>)  [unwired: 4 in, 1 out]
      }
      event "Move 10cm Left": Value Change {
        n151 = event-data() -> ()  [unwired: 1 in, 6 out]
        n152 = call "Joystick.vi"("Joystick"=FALSE, "Gantry In"=w442) -> ("Gantry Out"=w433:refnum<k24>)  [unwired: 8 in, 1 out]
        n153 = call "Move Inc.vi"("Axis"="X", "Speed"=25.0, "Distance"=-100.0, "Gantry In"=w433) -> ("Gantry Out"=w436:refnum<k24>)  [unwired: 6 in, 1 out]
      }
      event "Move 10cm Backward": Value Change {
        n154 = event-data() -> ()  [unwired: 1 in, 6 out]
        n155 = call "Joystick.vi"("Joystick"=FALSE, "Gantry In"=w453) -> ("Gantry Out"=w444:refnum<k24>)  [unwired: 8 in, 1 out]
        n156 = call "Move Inc.vi"("Axis"="Y", "Speed"=25.0, "Distance"=100.0, "Gantry In"=w444) -> ("Gantry Out"=w445:refnum<k24>)  [unwired: 6 in, 1 out]
      }
      event "Move 10cm Forward": Value Change {
        n157 = event-data() -> ()  [unwired: 1 in, 6 out]
        n158 = call "Joystick.vi"("Joystick"=FALSE, "Gantry In"=w464) -> ("Gantry Out"=w456:refnum<k24>)  [unwired: 8 in, 1 out]
        n159 = call "Move Inc.vi"("Axis"="Y", "Speed"=25.0, "Distance"=-100.0, "Gantry In"=w456) -> ("Gantry Out"=w455:refnum<k24>)  [unwired: 6 in, 1 out]
      }
      event "Move 10cm Right": Value Change {
        n160 = event-data() -> ()  [unwired: 1 in, 6 out]
        n161 = call "Joystick.vi"("Joystick"=FALSE, "Gantry In"=w475) -> ("Gantry Out"=w466:refnum<k24>)  [unwired: 8 in, 1 out]
        n162 = call "Move Inc.vi"("Axis"="X", "Speed"=25.0, "Distance"=100.0, "Gantry In"=w466) -> ("Gantry Out"=w467:refnum<k24>)  [unwired: 6 in, 1 out]
      }
      event "Dismount Silicon Tray": Value Change {
        n163 = event-data() -> ()  [unwired: 1 in, 6 out]
        n164 = Index Array(array=w486, index=1) -> (element=w483:i32)
        n165 = call-dynamic "Digital Write 1 Channel.vi"("Value"=FALSE, "Channel"=w483, "I-O.lvclass"=w484) -> ("I-O.lvclass 2"=w481:refnum<class "I-O.lvclass">)  [unwired: 7 in, 1 out]
      }
      event "Secure Silicon Tray": Value Change {
        n166 = event-data() -> ()  [unwired: 1 in, 6 out]
        n167 = Index Array(array=w495, index=1) -> (element=w493:i32)
        n168 = call-dynamic "Digital Write 1 Channel.vi"("Value"=TRUE, "Channel"=w493, "I-O.lvclass"=w496) -> ("I-O.lvclass 2"=w491:refnum<class "I-O.lvclass">)  [unwired: 7 in, 1 out]
      }
      event "Go": Value Change {
        n169 = event-data() -> ()  [unwired: 1 in, 6 out]
        n170 = for {
          tunnel: "XYZTheta" -> [w511] mode=indexing
          tunnel: [w509] -> w503 mode=indexing
          shift-right: [w507] -> w502
          shift-left: w504 -> [w508]
          i -> [w513]
          n171 = Equal To 0?(x=w511) -> (x = 0?=w512:bool)
          n172 = call "Get Current Position.vi"("Gantry In"=w508) -> ("XYZTheta Out"=w506:dbl[], "Gantry Out"=w507:refnum<k24>)  [unwired: 8 in, 1 out]
          n173 = Index Array(array=w506, index=w513) -> (element=w510:dbl)
          n174 = Select(t=w510, s=w512, f=w511) -> (s? t:f=w509:dbl)
        }
        n175 = call "ClearXYZTheta Go.vi"("XYZTheta In"=w503, "Gantry In"=w502) -> ("Gantry Out"=w497:refnum<k24>)  [unwired: 7 in, 2 out]
      }
      event "Z Go": Value Change {
        n176 = event-data() -> ()  [unwired: 1 in, 6 out]
        n177 = call "Z Go.vi"("Increment"=FALSE, "Return Immediately"=FALSE ("Increment"), "Speed In"=15.0 ("Speed"), "Position In"="Position", "Gantry In"=w523) -> ("Gantry Out"=w516:refnum<k24>)  [unwired: 3 in, 3 out]
      }
      event "Stop": Value Change {
        n178 = event-data() -> ()  [unwired: 1 in, 5 out]
        n179 = call "Joystick.vi"("Joystick"=FALSE, "Gantry In"=w531) -> ("Gantry Out"=w524:refnum<k24>)  [unwired: 8 in, 1 out]
      }
    }
  }
  n180 = Bundle By Name(cluster=w1, "Gantry"=w4, "I-O.lvclass"=w3) -> (w2:T7)
  n181 = Build Array(w7, w6, w8) -> (w12:dbl[][])
  n182 = call "Release Control Cluster.vi"("output cluster"=w2) -> ()  [unwired: 11 in]
  n183 = Transpose Matrix(1:w12) -> (0:w11:dbl[][])
  n184 = Open/Create/Replace File(operation (0:open)=T6."create") -> (refnum out=w10:refnum<file>)  [unwired: 5 in, 2 out]
  n185 = Array To Spreadsheet String(array=w11, 3:"%f" ("format string")) -> (spreadsheet string=w14:string)  [unwired: 1 in]
  n186 = Write to Text File(file (use dialog)=w10, text=w14) -> (refnum out=w13:refnum<file>)  [unwired: 2 in, 2 out]
  n187 = Close File(refnum=w13) -> ()  [unwired: 1 in, 2 out]
